vi "Set Query (attributes).vi"(8 "error in (no error)":errorcluster, 10 "Query":variant, 11 "URI in":refnum<class "URI.lvclass">) -> (0 "error out":errorcluster, 3 "URI out":refnum<class "URI.lvclass">)   [LabVIEW 2013, in "openURI.lvlib" / "URI.lvclass"]
doc: "The Query variant input must contain attributes of type \"string\".\nAll data contained in the variant will be ignored. All attributes that are not of type \"string\" will be ignored."
uses:
  URI.lvclass
  URI.lvclass/URI.ctl
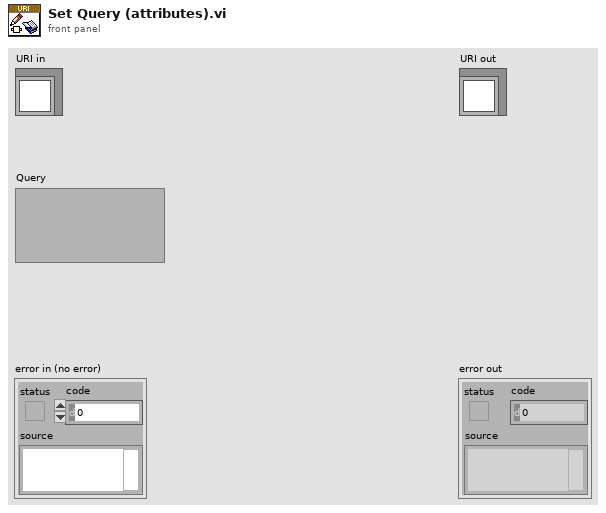
[diagram p1: front panel]
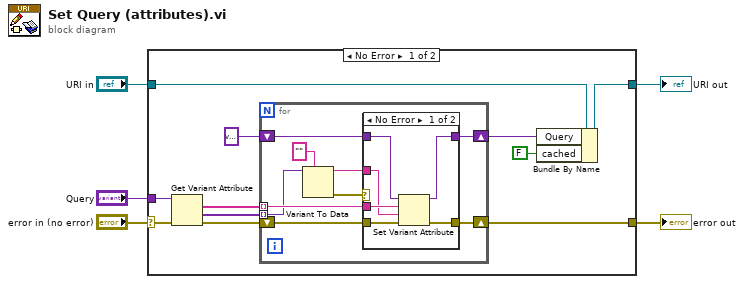
[diagram p0: block diagram]
diagram:
  n1 = case shown="No Error" "error in (no error)" {
    selector: "error in (no error)" -> [w10 w35]
    tunnel: [w13 w35] -> w4
    tunnel: [w15 w34] -> w2
    tunnel: "URI in" -> [w12 w34]
    tunnel: "Query" -> [w11 _]
    frame No Error {
      n2 = Get Variant Attribute(Variant=w11, error in=w10) -> (names=w8:string[], values=w7:variant[], error out=w9:errorcluster)  [unwired: 2 in, 1 out]
      n3 = for {
        shift-right: [w23] -> w13
        shift-left: w9 -> [w24]
        shift-right: [w25] -> w16
        shift-left: variant ("Query") -> [w22]
        tunnel: w8 -> [w21] mode=indexing
        tunnel: w7 -> [w20] mode=indexing
        n4 = Variant To Data(type="", Variant=w20) -> (data=w17:string, error out=w19:errorcluster)  [unwired: 1 in]
        n5 = case shown="No Error" w19 {
          tunnel: [w31 w33] -> w25
          tunnel: w24 -> [w30 w32]
          tunnel: [w29 w32] -> w23
          tunnel: w22 -> [w28 w33]
          tunnel: w21 -> [w27 _]
          tunnel: w17 -> [w26 _]
          frame No Error {
            n6 = Set Variant Attribute(Variant=w28, name=w27, value=w26, error in=w30) -> (Variant out=w31:variant, error out=w29:errorcluster)  [unwired: 1 out]
          }
          frame Error {
          }
        }
      }
      n7 = Bundle By Name(cluster=w12, "Query"=w16, "cached"=FALSE) -> (w15:refnum<class "URI.lvclass">)
    }
    frame Error {
    }
  }
  "error out" <- w4
  "URI out" <- w2
